vi "close.vi"(8 "error in":errorcluster, 11 "UI Reference runtime in":refnum<class "UI Reference runtime.lvclass">) -> (0 "error out":errorcluster)   [LabVIEW 2013, in "UI Reference runtime.lvclass"]
doc: "Provides an interface for terminating a module instance. While this interface performs no operations, a child should close and deallocate any open references or memory."
uses:
  UI Reference runtime.lvclass
  UI Reference runtime.lvclass/UI Reference runtime.ctl
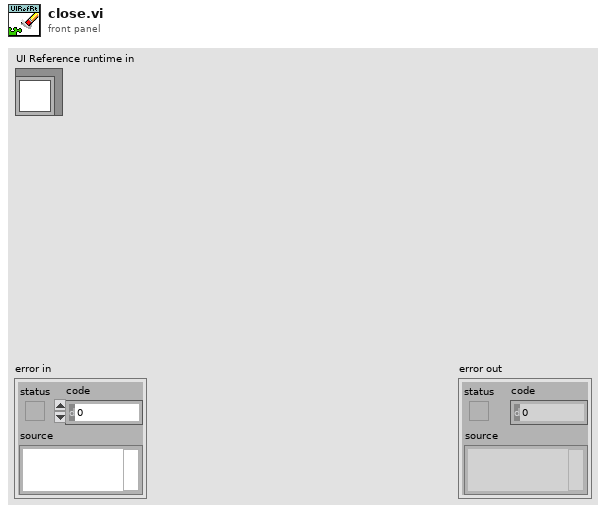
[diagram p1: front panel]
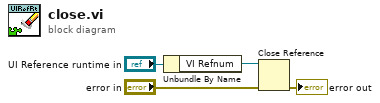
[diagram p0: block diagram]
diagram:
  n1 = Unbundle By Name("UI Reference runtime in") -> ("VI Refnum"=w1:refnum<vi>)
  n2 = Close Reference(reference=w1, error in (no error)="error in") -> (error out=→"error out":errorcluster)
